vi "Send Event.vi"(10 "Data":variant, 11 "DAQmx Shortcut":T1) -> ()   [LabVIEW 2019, in "DAQmx.lvlib" / "DAQmx.lvclass"]
uses:
  DAQmx.lvclass
  DAQmx Shortcut.ctl
  Packed Libraries/Messaging.lvlibp/Message Cluster.ctl
  Packed Libraries/Messaging.lvlibp
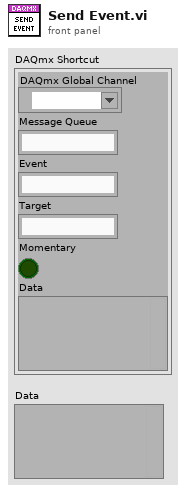
[diagram p1: front panel]
types:
  T1 = typedef "DAQmx.lvlib/DAQmx.lvclass/DAQmx Shortcut.ctl" = cluster{"DAQmx Global Channel":refnum<k21>, "Message Queue":string, "Event":string, "Target":string, "Momentary":bool, "Data":variant}
  T2 = typedef "Messaging.lvlibp/Message Cluster.ctl" = cluster{"Event":string, "Source":string, "Target":string, "Data":variant}
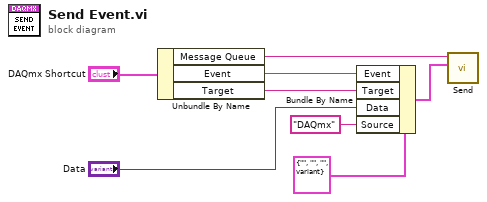
[diagram p0: block diagram]
diagram:
  n1 = Unbundle By Name("DAQmx Shortcut") -> ("Message Queue"=w8:string, "Event"=w5:string, "Target"=w4:string)
  n2 = Bundle By Name(cluster=T2 {"Event"="", "Source"="", "Target"="", "Data"=variant} ("Message"), "Event"=w5, "Target"=w4, "Data"="Data", "Source"="DAQmx") -> (w6:T2)
  n3 = call "Send.vi"("Message"=w6, "Queue Name"=w8) -> ()  [unwired: 9 in, 1 out]
